vi "Select Device.vi"(8 "error in (no error)":errorcluster, 10 "Device":refnum<class "Device.lvclass">, 11 "picoG in":refnum<class "picoG.lvclass">) -> (0 "error out":errorcluster, 3 "picoG out":refnum<class "picoG.lvclass">)   [LabVIEW 2020, in "PicoG-App.lvlib" / "picoG.lvclass"]
uses:
  picoG.lvclass
  Device/Device.lvclass
  picoG.lvclass/picoG.ctl
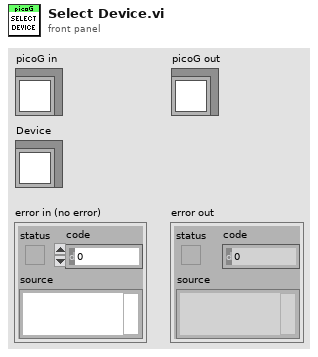
[diagram p1: front panel]
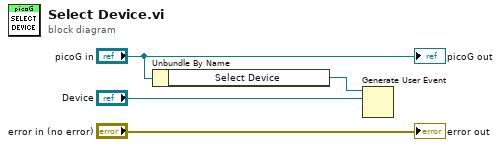
[diagram p0: block diagram]
diagram:
  n1 = Unbundle By Name("picoG in") -> ("Select Device"=w2:refnum<user-event>)
  n2 = Generate User Event(user event=w2, event data cluster="Device") -> ()  [unwired: 2 in, 2 out]
  "error out" <- "error in (no error)"
  "picoG out" <- "picoG in"
